vi "Load Document.vi"(0 "Spreadsheet In":refnum<class "Spreadsheet.lvclass">, 1 "Path":path, 5 "error in (no error)":errorcluster) -> (14 "Spreadsheet Out":refnum<class "Spreadsheet.lvclass">, 15 "xml":string, 19 "error out":errorcluster)   [LabVIEW 2014, in "Spreadsheet.lvclass"]
uses:
  Spreadsheet.lvclass
  XML/DOMDefRefCommand.ctl
  XML/Public XML/RowDataFilter.ctl
  Spreadsheet.lvclass/Spreadsheet.ctl
  Document_class/Document.lvclass
  XML.lvlib
  <resource>/objmgr/DOMUserDefRef.rc
panel:
  out "Tables":i32 caption="Of"
  out "Table":i32
  # "Local"
  # "Input"
  # "Output"
  # "number-columns-repeated=12\nvalue-type=\"string\"\n<text:p xmlns:text=\"urn:oasis:names:tc:opendocument:xmlns:text:1.0\">Title1</text:p>"
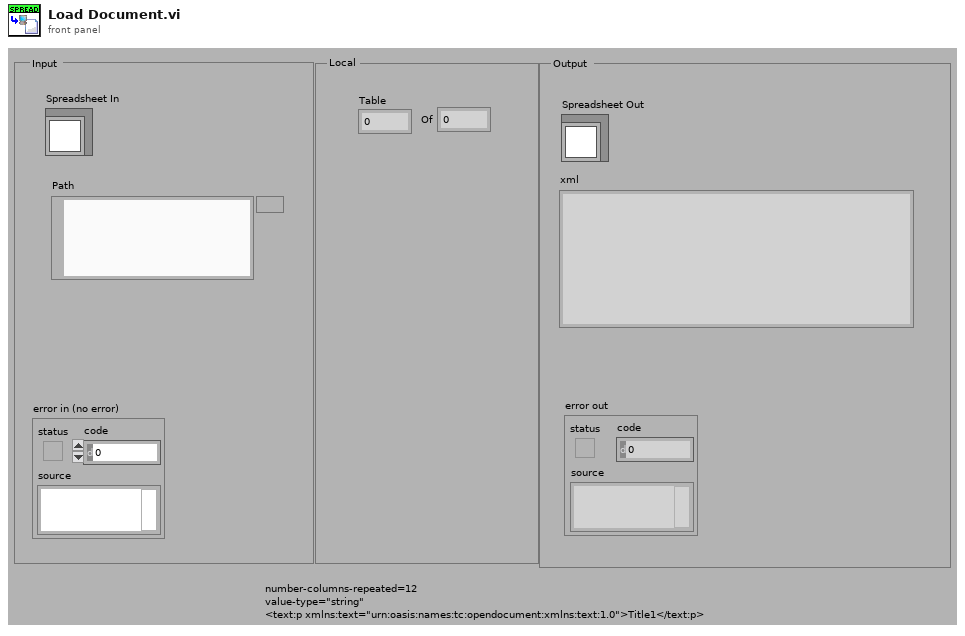
[diagram p1: front panel]
types:
  T1 = typedef "DOMDefRefCommand.ctl" = enum16{"No Command - Error", "Initialise", "Open Document", "Allocate RefNum", "Close Document"}
  T2 = cluster{"Table Data":string[][], "Cell Info":string[][], "SheetName":string}
  T3 = typedef "RowDataFilter.ctl" = enum16{"No Filter - Error", "Row Values", "Row Data", "#Rows Repeated", "#Columns Repeated"}
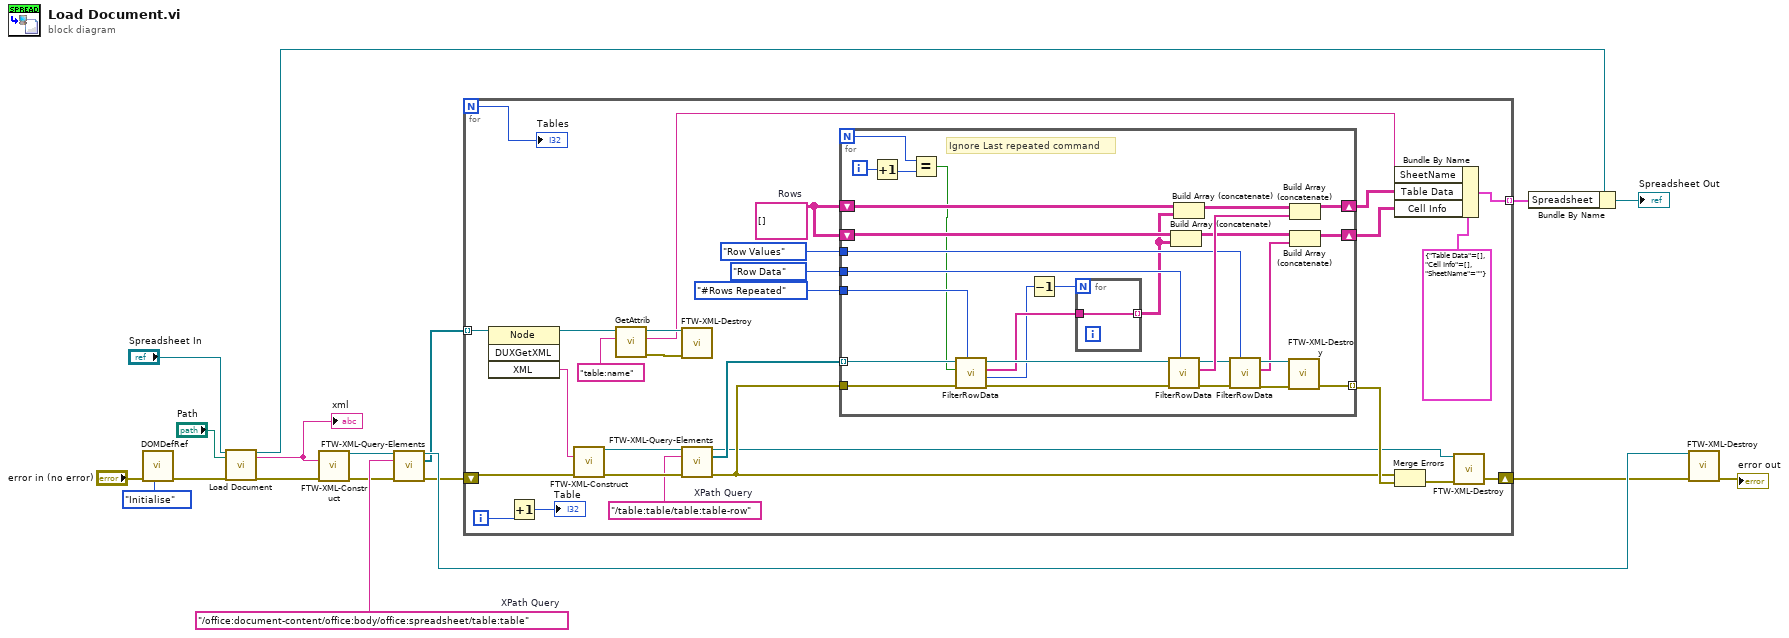
[diagram p0: block diagram]
diagram:
  w11 = "/office:document-content/office:body/office:spreadsheet/table:table"  # XPath Query
  n1 = call "DOMDefRef.vi"("DOMUserDefRefCommand"=DOMDefRefCommand."Initialise", "error in (no error)"="error in (no error)") -> ("error out"=w1:errorcluster)  [unwired: 4 in, 2 out]
  n2 = call-parent "Load Document.vi"("Document In"="Spreadsheet In", "Path"="Path", "error in (no error)"=w1) -> ("Document Out"=w16:refnum<class "Spreadsheet.lvclass">, "xml"=w12:string, "error out"=w13:errorcluster)  [unwired: 14 in]
  "xml" <- w12
  n3 = call "FTW-XML-Construct.vi"("XML String"=w12, "error in"=w13) -> ("XML Document"=w7:refnum<k20>, "error out"=w8:errorcluster)  [unwired: 12 in]
  n4 = call "FTW-XML-Query-Elements.vi"("XML Node"=w7, "XPath Query"=w11, "error in"=w8) -> ("XML Node out"=w10:refnum<k20>, "Matching Nodes"=w6:refnum<k20>[], "error out"=w5:errorcluster)  [unwired: 9 in, 1 out]
  n5 = for {
    N -> [w20]
    tunnel: w6 -> [w36] mode=indexing
    shift-right: [w37] -> w9
    shift-left: w5 -> [w35]
    tunnel: [w39] -> w4 mode=indexing
    i -> [w21]
    w30 = "/table:table/table:table-row"  # XPath Query
    w43 = string[][] []  # Rows
    n6 = invoke class="Node" method="DUXGetXML"(reference=w36) -> (reference out=w26:refnum<k20>, "XML"=w34:string)  [unwired: 3 in, 2 out]
    n7 = Increment(x=w21) -> (x+1=→"Table":i32)
    n8 = call "FTW-XML-Construct.vi"("XML String"=w34, "error in"=w35) -> ("XML Document"=w33:refnum<k20>, "error out"=w32:errorcluster)  [unwired: 12 in]
    n9 = call "GetAttrib.vi"("Attrib"="table:name" ("XPath Query"), "Refnum in"=w26) -> ("error out"=w24:errorcluster, "Value"=w23:string, "Refnum out"=w25:refnum<k20>)  [unwired: 7 in]
    n10 = call "FTW-XML-Destroy.vi"("XML Node"=w25, "error in"=w24) -> ()  [unwired: 13 in, 1 out]
    n11 = call "FTW-XML-Query-Elements.vi"("XML Node"=w33, "XPath Query"=w30, "error in"=w32) -> ("XML Node out"=w28:refnum<k20>, "Matching Nodes"=w29:refnum<k20>[], "error out"=w31:errorcluster)  [unwired: 9 in, 1 out]
    n12 = for {
      N -> [w49]
      tunnel: w29 -> [w74] mode=indexing
      tunnel: w31 -> [w73]
      tunnel: [w72] -> w46 mode=indexing
      tunnel: RowDataFilter."#Rows Repeated" ("Row Filter") -> [w71]
      shift-right: [w67] -> w41
      shift-left: w43 -> [w56]
      tunnel: RowDataFilter."Row Data" ("Row Filter") -> [w68]
      shift-right: [w65] -> w40
      shift-left: w43 -> [w58]
      tunnel: RowDataFilter."Row Values" ("Row Filter") -> [w60]
      i -> [w51]
      # "Ignore Last repeated command"
      n13 = Increment(x=w51) -> (x+1=w50:i32)
      n14 = Equal?(x=w49, y=w50) -> (x = y?=w48:bool)
      n15 = call "FilterRowData.vi"("Row Filter"=w71, "error in (no error)"=w73, "Ignore?"=w48, "Row XML Node"=w74) -> ("error out"=w70:errorcluster, "Number Out"=w53:i32, "Row Data"=w54:string[], "XML Node Out"=w69:refnum<k20>)  [unwired: 1 in]
      n16 = Decrement(x=w53) -> (x-1=w47:i32)
      n17 = for {
        N: w47 -> [_]
        tunnel: w54 -> [w75]
        tunnel: [w75] -> w52 mode=indexing
      }
      n18 = call "FilterRowData.vi"("Row Filter"=w68, "error in (no error)"=w70, "Row XML Node"=w69) -> ("error out"=w64:errorcluster, "Row Data"=w66:string[], "XML Node Out"=w63:refnum<k20>)  [unwired: 2 in, 1 out]
      n19 = Build Array (concatenate)(w58, w52) -> (w57:string[][])
      n20 = Build Array (concatenate)(w56, w52) -> (w55:string[][])
      n21 = call "FilterRowData.vi"("Row Filter"=w60, "error in (no error)"=w64, "Row XML Node"=w63) -> ("error out"=w61:errorcluster, "Row Data"=w59:string[], "XML Node Out"=w62:refnum<k20>)  [unwired: 2 in, 1 out]
      n22 = call "FTW-XML-Destroy.vi"("XML Node"=w62, "error in"=w61) -> ("error out"=w72:errorcluster)  [unwired: 13 in]
      n23 = Build Array (concatenate)(w55, w66) -> (w67:string[][])
      n24 = Build Array (concatenate)(w57, w59) -> (w65:string[][])
    }
    n25 = Bundle By Name(cluster=T2 {"Table Data"=[], "Cell Info"=[], "SheetName"=""} ("Sheet"), "SheetName"=w23, "Table Data"=w41, "Cell Info"=w40) -> (w39:T2)
    n26 = Merge Errors(w31, w46) -> (w38:errorcluster)
    n27 = call "FTW-XML-Destroy.vi"("XML Node"=w28, "error in"=w38) -> ("error out"=w37:errorcluster)  [unwired: 13 in]
    "Tables" <- w20
  }
  n28 = Bundle By Name(cluster=w16, "Spreadsheet"=w4) -> (→"Spreadsheet Out":refnum<class "Spreadsheet.lvclass">)
  n29 = call "FTW-XML-Destroy.vi"("XML Node"=w10, "error in"=w9) -> ("error out"=→"error out":errorcluster)  [unwired: 13 in]
